vi "GetPixelData.vi"   [LabVIEW 2019]
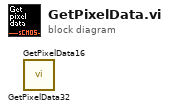
[diagram p0: block diagram]
diagram:
  n1 = call <userlib>:"GetPixelData32.vi"() -> ()  [unwired: 17 in, 3 out]
  n2 = call <userlib>:"GetPixelData16.vi"() -> ()  [unwired: 17 in, 3 out]
